vi "Actor Core.vi"(8 "error in":errorcluster, 11 "State in":refnum<class "Connect Command.lvclass">) -> (0 "error out":errorcluster, 3 "Actor out":refnum<class "Actor.lvclass">)   [LabVIEW 2013, in "Receiver.lvlib" / "Receiver Commands Using Processor.lvlib" / "Connect Command.lvlib" / "Connect Command.lvclass"]
doc: "(<B>Filename</B>: Actor Framework.lvlib:Actor.lvclass:Actor Core.vi)\n\nThis override invokes Entry.vi on the initial state, prior to calling the parent Actor Core. Adding this behavior to Actor Core (instead of an override of Pre Launch Init.vi) allows the initial state to launch a nested actor as part of its entry behavior.\n\nReceives messages to the actor, reacts to them, and initiates any error handling that may shut the actor down.\n\nDescendant classes may override this VI to append parallel tasks for the actor to complete while it handles messages. Overrides use the Call Parent Method node."
uses:
  Connect Command.lvclass
  <vilib>/ActorFramework/Actor/Actor.lvclass
  Command Processor/Command/Command Status.ctl
  Command Processor/Command/State Status.ctl
  Receiver Command.lvclass
  Command Processor/Command/Command.lvclass
panel:
  in  "Command Status":T1
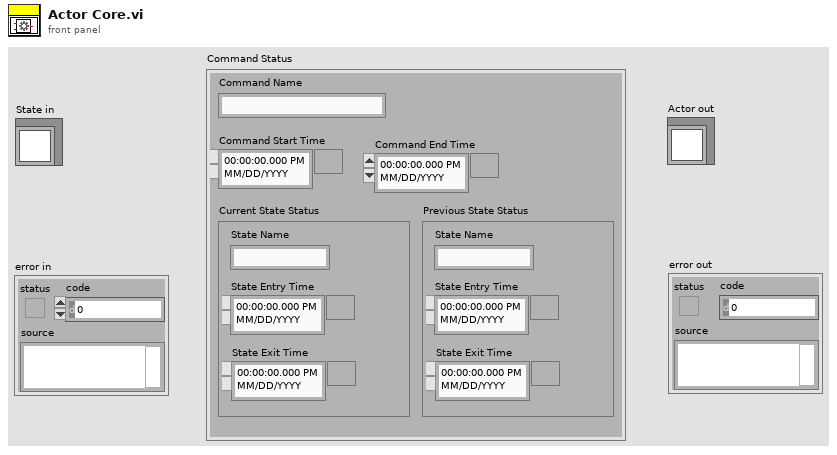
[diagram p1: front panel]
types:
  T1 = typedef "Command Processor.lvlib/Command.lvlib/Command.lvclass/Command Status.ctl" = cluster{"Command Name":string, "Current State Status":T2, "Command Start Time":timestamp, "Command End Time":timestamp, "Previous State Status":T2}
  T2 = typedef "Command Processor.lvlib/Command.lvlib/Command.lvclass/State Status.ctl" = cluster{"State Name":string, "State Entry Time":timestamp, "State Exit Time":timestamp}
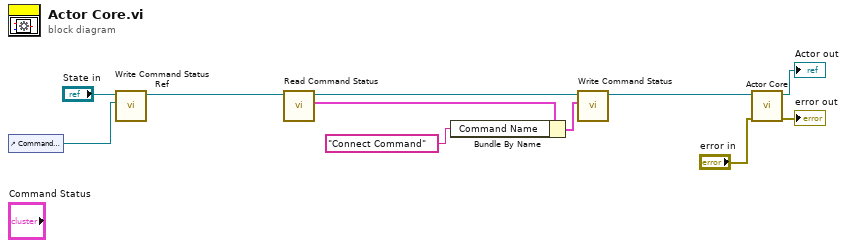
[diagram p0: block diagram]
diagram:
  n1 = control-ref of="Command Status"() -> (w2:refnum<vi>)
  n2 = call-dynamic "Write Command Status Ref.vi"("Command Status Ref"=w2, "Command in"="State in") -> ("Command out"=w1:refnum<class "Connect Command.lvclass">)  [unwired: 8 in, 1 out]
  n3 = call-dynamic "Read Command Status.vi"("Command in"=w1) -> ("Command Status"=w6:T1, "Command out"=w7:refnum<class "Connect Command.lvclass">)  [unwired: 8 in, 1 out]
  n4 = Bundle By Name(cluster=w6, "Command Name"="Connect Command" ("Name")) -> (w5:T1)
  n5 = call-dynamic "Write Command Status.vi"("Command Status"=w5, "Command in"=w7) -> ("Command out"=w8:refnum<class "Connect Command.lvclass">)  [unwired: 8 in, 1 out]
  n6 = call-parent "Actor Core.vi"("error in"="error in", "State in"=w8) -> ("error out"=→"error out":errorcluster, "Actor out"=→"Actor out":refnum<class "Actor.lvclass">)  [unwired: 8 in]
